vi "Configure.vi"(8 "error in":errorcluster, 10 "Output Settings":T1={"Voltage (V)"=1.0} {"Voltage (V)" min=-424.2 max=424.2 step=1.0 format="%#.1f"}, 11 "Instrument Driver in":refnum<class "Instrument Driver.lvclass">) -> (0 "error out":errorcluster, 3 "Instrument Driver out":refnum<class "Instrument Driver.lvclass">)   [LabVIEW 2020, in "Plugin Instrument Driver.lvlib" / "Instrument Driver.lvclass"]
doc: "This VI Configures the output channel."
uses:
  Instrument Driver.lvclass
  Typedefs/Output Settings.ctl
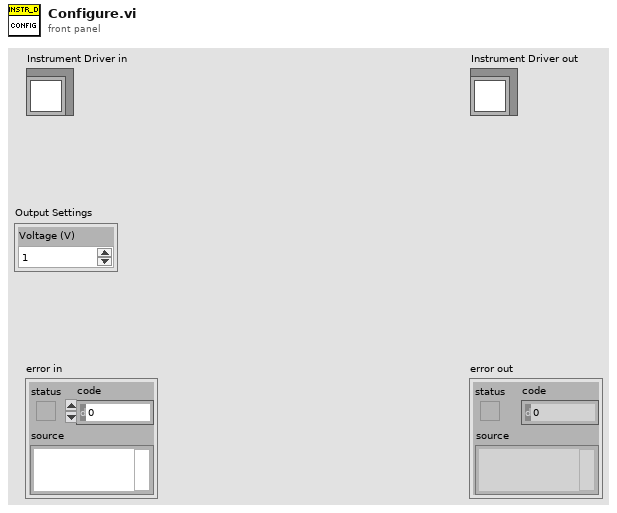
[diagram p1: front panel]
types:
  T1 = typedef "Plugin Instrument Driver.lvlib/Instrument Driver.lvclass/Output Settings.ctl" = cluster{"Voltage (V)":dbl}
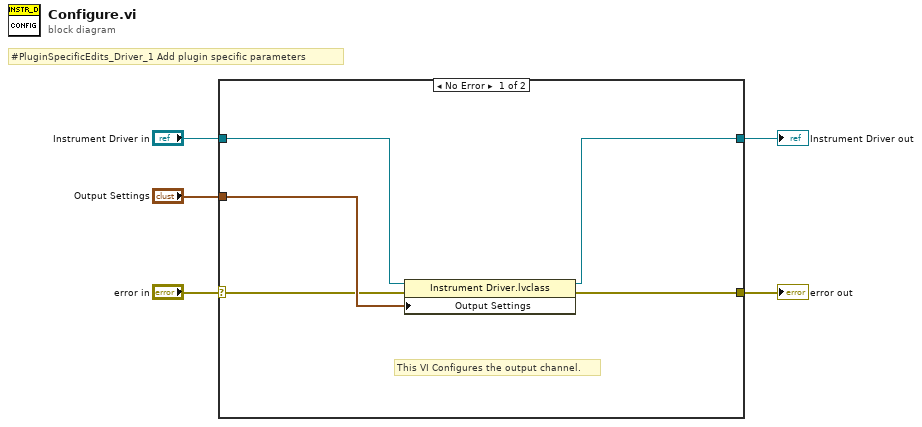
[diagram p0: block diagram]
diagram:
  # "#PluginSpecificEdits_Driver_1 Add plugin specific parameters"
  n1 = case shown="No Error" "error in" {
    selector: "error in" -> [w7 w12]
    tunnel: [w6 w12] -> w4
    tunnel: [w9 w11] -> w2
    tunnel: "Instrument Driver in" -> [w10 w11]
    tunnel: "Output Settings" -> [w8 _]
    frame No Error {
      # "This VI Configures the output channel."
      n2 = property class="Instrument Driver.lvclass"(reference=w10, error in=w7, "Output Settings"=w8) -> (reference out=w9:refnum<class "Instrument Driver.lvclass">, error out=w6:errorcluster)
    }
    frame Error {
    }
  }
  "error out" <- w4
  "Instrument Driver out" <- w2
